vi "MAC_computerId_get.vi"() -> (0 "error out":errorcluster, 1 "return code":i32, 3 "standard output":string)   [LabVIEW 2018]
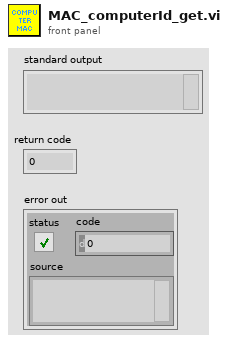
[diagram p1: front panel]
types:
  T1 = enum32{"invalid app kind", "Development System", "Run Time System", "Student Edition", "Embedded LabVIEW", "Evaluation", "Custom"}
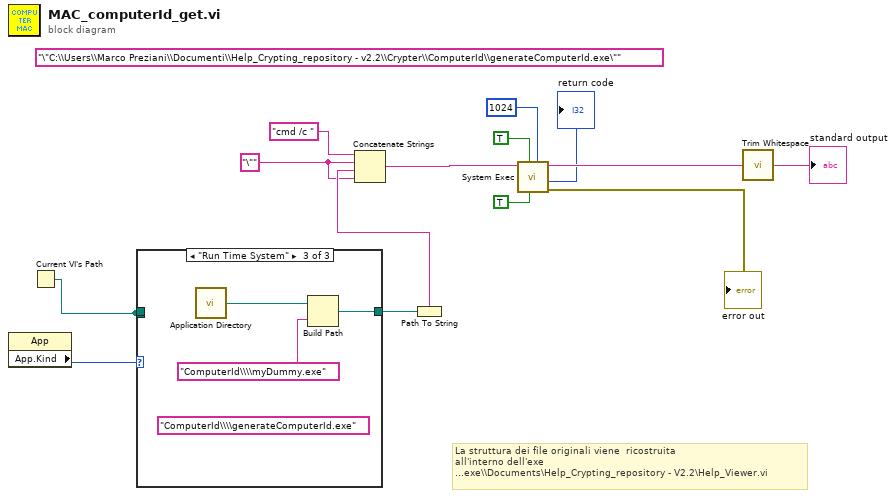
[diagram p0: block diagram]
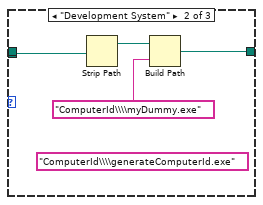
[diagram p3: hidden frame]
diagram:
  w2 = "\"" ("string")
  (unwired) "\"C:\\Users\\Marco Preziani\\Documenti\\Help_Crypting_repository - v2.2\\Crypter\\ComputerId\\generateComputerId.exe\""
  # "La struttura dei file originali viene  ricostruita\nall'interno dell'exe\n...exe\\\\Documents\\Help_Crypting_repository - V2.2\\Help_Viewer.vi"
  n1 = property class="App"() -> ("App.Kind"=w6:T1)  [unwired: 2 in, 2 out]
  n2 = Current VI's Path() -> (path=w4:path)
  n3 = case shown="\"Run Time System\"" w6 {
    tunnel: w4 -> [_ w19 _]
    tunnel: [w15 w17 w21] -> w5
    tunnel: w4 -> [w15 _ _]
    frame "invalid app kind", Default {
    }
    frame "Development System" {
      (unwired) "ComputerId\\\\generateComputerId.exe" ("name or relative path")
      n4 = Strip Path(path=w19) -> (stripped path=w18:path)  [unwired: 1 out]
      n5 = Build Path(base path=w18, name or relative path="ComputerId\\\\myDummy.exe") -> (appended path=w17:path)
    }
    frame "Run Time System" {
      (unwired) "ComputerId\\\\generateComputerId.exe" ("name or relative path")
      n6 = call <vilib>:"Application Directory.vi"() -> ("Application Directory"=w20:path)
      n7 = Build Path(base path=w20, name or relative path="ComputerId\\\\myDummy.exe") -> (appended path=w21:path)
    }
  }
  n8 = Path To String(path=w5) -> (string=w3:string)
  n9 = Concatenate Strings("cmd /c " ("string"), w2, w3, w2) -> (w13:string)
  n10 = call <vilib>:"System Exec.vi"("expected output size  (4096)"=u32 1024, "run minimized? (F)"=TRUE, "wait until completion? (T)"=TRUE, "command line"=w13) -> ("error out"=→"error out":errorcluster, "return code"=→"return code":i32, "standard output"=w14:string)  [unwired: 4 in, 1 out]
  n11 = call <vilib>:"Trim Whitespace.vi"("string"=w14) -> ("trimmed string"=→"standard output":string)  [unwired: 1 in]
